vi "0037-0005_SHT31.vi"() -> ()   [LabVIEW 2014]
panel:
  in  "GPIO":u8
  out "x = y?":bool
  out "湿度":dbl format="%.2g"
  out "温度":dbl format="%.2g"
  in  "停止ボタン":bool
  # "℃"
  # "％RH"
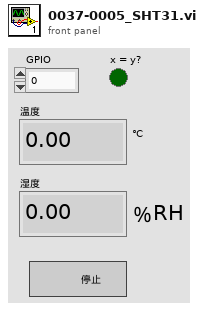
[diagram p1: front panel]
types:
  T1 = cluster{"bitRate":u32, "address":u8, "autoReadRespond":bool, "writeTimeout":u16, "readTimeout":u16, "sclLowTimeout":bool, "transferRetries":u16}
  T2 = typedef "CP2112_device.ctl" = i32
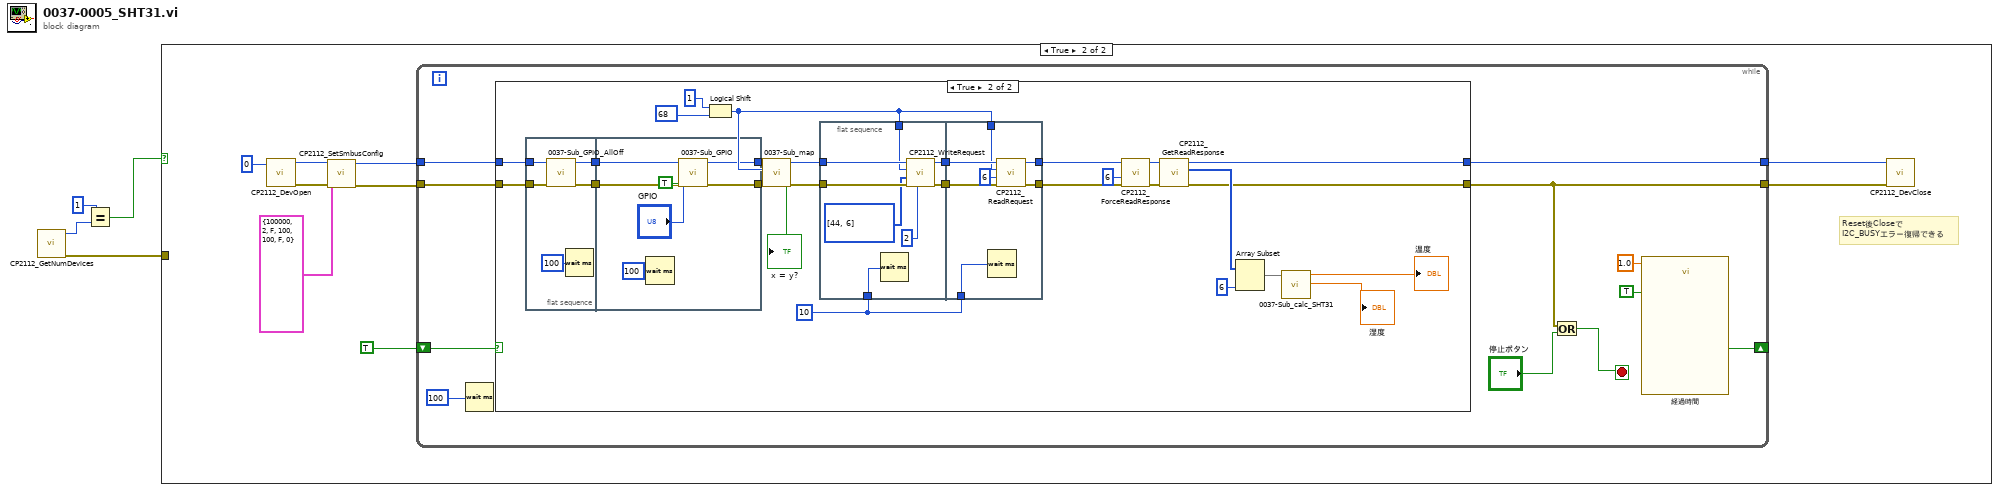
[diagram p0: block diagram]
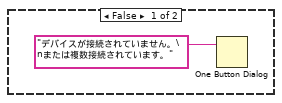
[diagram p2: hidden frame]
diagram:
  n1 = call "CP2112_GetNumDevices.vi"() -> ("error out"=w1:errorcluster, "numDevices"=w3:i32)  [unwired: 9 in, 1 out]
  n2 = Equal?(x=1, y=w3) -> (x = y?=w2:bool)
  n3 = case shown="TRUE" w2 {
    tunnel: w1 -> [_ _]
    frame False {
      n4 = One Button Dialog(message="デバイスが接続されていません。\nまたは複数接続されています。" ("メッセージ")) -> ()  [unwired: 1 in, 1 out]
    }
    frame True {
      # "Reset後Closeで\nI2C_BUSYエラー復帰できる"
      n5 = call "CP2112_DevOpen.vi"("deviceNum"=0) -> ("error out"=w9:errorcluster, "device"=w10:T2)  [unwired: 8 in, 1 out]
      n6 = call "CP2112_SetSmbusConfig.vi"("error in (no error)"=w9, "smbusInfo"=T1 {"bitRate"=100000, "address"=2, "autoReadRespond"=FALSE, "writeTimeout"=100, "readTimeout"=100, "sclLowTimeout"=FALSE, "transferRetries"=0}, "device"=w10) -> ("error out"=w11:errorcluster, "deviceOut"=w12:T2)  [unwired: 6 in, 1 out]
      n7 = while {
        tunnel: w11 -> [w25]
        tunnel: w12 -> [w24]
        tunnel: [w21] -> w7
        tunnel: [w20] -> w6
        shift-right: [w17] -> _
        shift-left: TRUE ("Auto Reset") -> [w18]
        stop <- w22 stop-if-true
        n8 = Wait (ms)(milliseconds to wait=u32 100 ("ミリ秒待機時間")) -> ()  [unwired: 1 out]
        n9 = case shown="TRUE" w18 {
          tunnel: w25 -> [w26 w35]
          tunnel: w24 -> [w27 w36]
          tunnel: [w26 w38] -> w21
          tunnel: [w27 w37] -> w20
          frame False {
          }
          frame True {
            w42 = u32 10 ("ミリ秒待機時間")
            n10 = flat-sequence {
              tunnel: w35 -> [w57]
              tunnel: w36 -> [w56]
              tunnel: [w59] -> w29
              tunnel: [w58] -> w28
              tunnel: [w66] -> w34
              tunnel: [w65] -> w33
              tunnel: w29 -> [w61]
              tunnel: w28 -> [w60]
              frame #0 {
                n11 = call "0037-Sub_GPIO_AllOff.vi"("エラー出力 2"=w57, "device"=w56) -> ("エラー出力"=w58:errorcluster, "deviceOut"=w59:T2)  [unwired: 8 in]
                n12 = Wait (ms)(milliseconds to wait=u32 100 ("ミリ秒待機時間")) -> ()  [unwired: 1 out]
              }
              frame #1 {
                n13 = Wait (ms)(milliseconds to wait=u32 100 ("ミリ秒待機時間")) -> ()  [unwired: 1 out]
                n14 = call "0037-Sub_GPIO.vi"("エラー出力 2"=w60, "ブール"=TRUE, "GPIO"="GPIO", "device"=w61) -> ("エラー出力"=w65:errorcluster, "deviceOut"=w66:T2)  [unwired: 6 in]
              }
            }
            n15 = Logical Shift(y=1, x=68) -> (x << y=w30:i32)
            n16 = call "0037-Sub_map.vi"("error out"=w33, "アドレス"=w30, "device"=w34) -> ("error out 2"=w41:errorcluster, "x = y?"=→"x = y?":bool, "device 2"=w40:T2)  [unwired: 5 in]
            n17 = flat-sequence {
              tunnel: w41 -> [w74]
              tunnel: w40 -> [w73]
              tunnel: w30 -> [w68]
              tunnel: [w72] -> w46
              tunnel: [w71] -> w45
              tunnel: w42 -> [w67]
              tunnel: w46 -> [w79]
              tunnel: w45 -> [w78]
              tunnel: [w80] -> w44
              tunnel: [w77] -> w43
              tunnel: w30 -> [w76]
              tunnel: w42 -> [w75]
              frame #0 {
                n18 = Wait (ms)(milliseconds to wait=w67) -> ()  [unwired: 1 out]
                n19 = call "CP2112_WriteRequest.vi"("numBytesToWrite"=i16 2 ("numByteToRead"), "error in (no error)"=w74, "buffer"=u8[] [44, 6], "slaveAddress"=w68, "device"=w73) -> ("error out"=w72:errorcluster, "deviceOut"=w71:T2)  [unwired: 4 in, 1 out]
              }
              frame #1 {
                n20 = Wait (ms)(milliseconds to wait=w75) -> ()  [unwired: 1 out]
                n21 = call "CP2112_ReadRequest.vi"("error in (no error)"=w79, "numByteToRead"=i16 6, "slaveAddress"=w76, "device"=w78) -> ("error out"=w80:errorcluster, "deviceOut"=w77:T2)  [unwired: 5 in, 1 out]
              }
            }
            n22 = call "CP2112_ForceReadResponse.vi"("error in (no error)"=w44, "numByteToRead"=i16 6, "device"=w43) -> ("error out"=w54:errorcluster, "deviceOut"=w53:T2)  [unwired: 6 in, 1 out]
            n23 = call "CP2112_GetReadResponse.vi"("error in (no error)"=w54, "device"=w53) -> ("error out"=w38:errorcluster, "buffer"=w50:u8[], "deviceOut"=w37:T2)  [unwired: 4 in, 3 out]
            n24 = Array Subset(array=w50, length=6 ("長さ")) -> (w52:u8[])  [unwired: 1 in]
            n25 = call "0037-Sub_calc_SHT31.vi"("Data"=w52) -> ("数値"=→"湿度":dbl, "数値 2"=→"温度":dbl)  [unwired: 9 in]
          }
        }
        n26 = Or(x=w21, y="停止ボタン") -> (x .or. y?=w22:bool)
        n27 = call "経過時間"("Time Target (s)"=1.0, "Auto Reset"=TRUE) -> ("Time has Elapsed"=w17:bool)  [unwired: 10 in, 7 out]
      }
      n28 = call "CP2112_DevClose.vi"("error in (no error)"=w7, "device"=w6) -> ()  [unwired: 9 in, 1 out]
    }
  }
